vi "Handle Exception.vi"(7 "Inputs":T2, 8 "error in (no error)":errorcluster, 11 "WebSocket Handler in":refnum<class "WebSocket Handler.lvclass">) -> (0 "error out":errorcluster, 5 "Outputs":T1)   [LabVIEW 2020, in "HTTP Server.lvlib" / "WebSocket Handler.lvclass"]
uses:
  WebSocket Handler.lvclass
  Exception Inputs.ctl
  <vilib>/IlluminatedG/IG HTTP Utils/HTTP Utils/Response/Response.lvclass
  Arguments/Arguments.lvclass
  <vilib>/IlluminatedG/IG HTTP Utils/HTTP Utils/Request/Request.lvclass
  <vilib>/IlluminatedG/lv-stream/URI/URI.lvclass
  Session/Session.lvclass
  Exception Outputs.ctl
  HTTP Server.lvlib
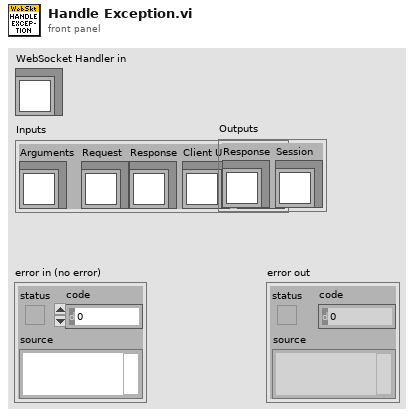
[diagram p1: front panel]
types:
  T1 = typedef "HTTP Server.lvlib/Exception Outputs.ctl" = cluster{"Response":refnum<class "Response.lvclass">, "Session":refnum<class "Session.lvclass">}
  T2 = typedef "HTTP Server.lvlib/Exception Inputs.ctl" = cluster{"Arguments":refnum<class "Arguments.lvclass">, "Request":refnum<class "Request.lvclass">, "Response":refnum<class "Response.lvclass">, "Client URI":refnum<class "URI.lvclass">, "Session":refnum<class "Session.lvclass">}
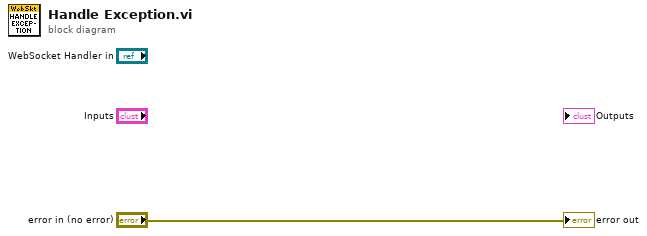
[diagram p0: block diagram]
diagram:
  "error out" <- "error in (no error)"
